vi "Helium Test - Step 5.vi"(7 "Step":i32, 8 "error in":errorcluster, 9 "Test Results In":T9, 10 "Gas":T8, 11 "Test Configuration":T1) -> (0 "error out":errorcluster, 1 "Test Results Out":T9, 2 "Gas Out":T8 caption="Gas", 3 "Test Configuration Out":T1)   [LabVIEW 2015]
uses:
  CAN Communication/PAS/Typedefs/Session Handle.ctl
  CAN Communication/PAS/PAS.lvclass
  Controls/Test Results.ctl
  Controls/Step Result.ctl
  Controls/Test Configuration.ctl
  Controls/Vacuum Test.ctl
  Controls/Test Timing.ctl
  Controls/Vaccum Thresholds.ctl
  Controls/Helium Test.ctl
  Controls/Helium Thresholds.ctl
  Controls/Functional Test.ctl
  CAN Communication/PAS/Typedefs/Valves.ctl
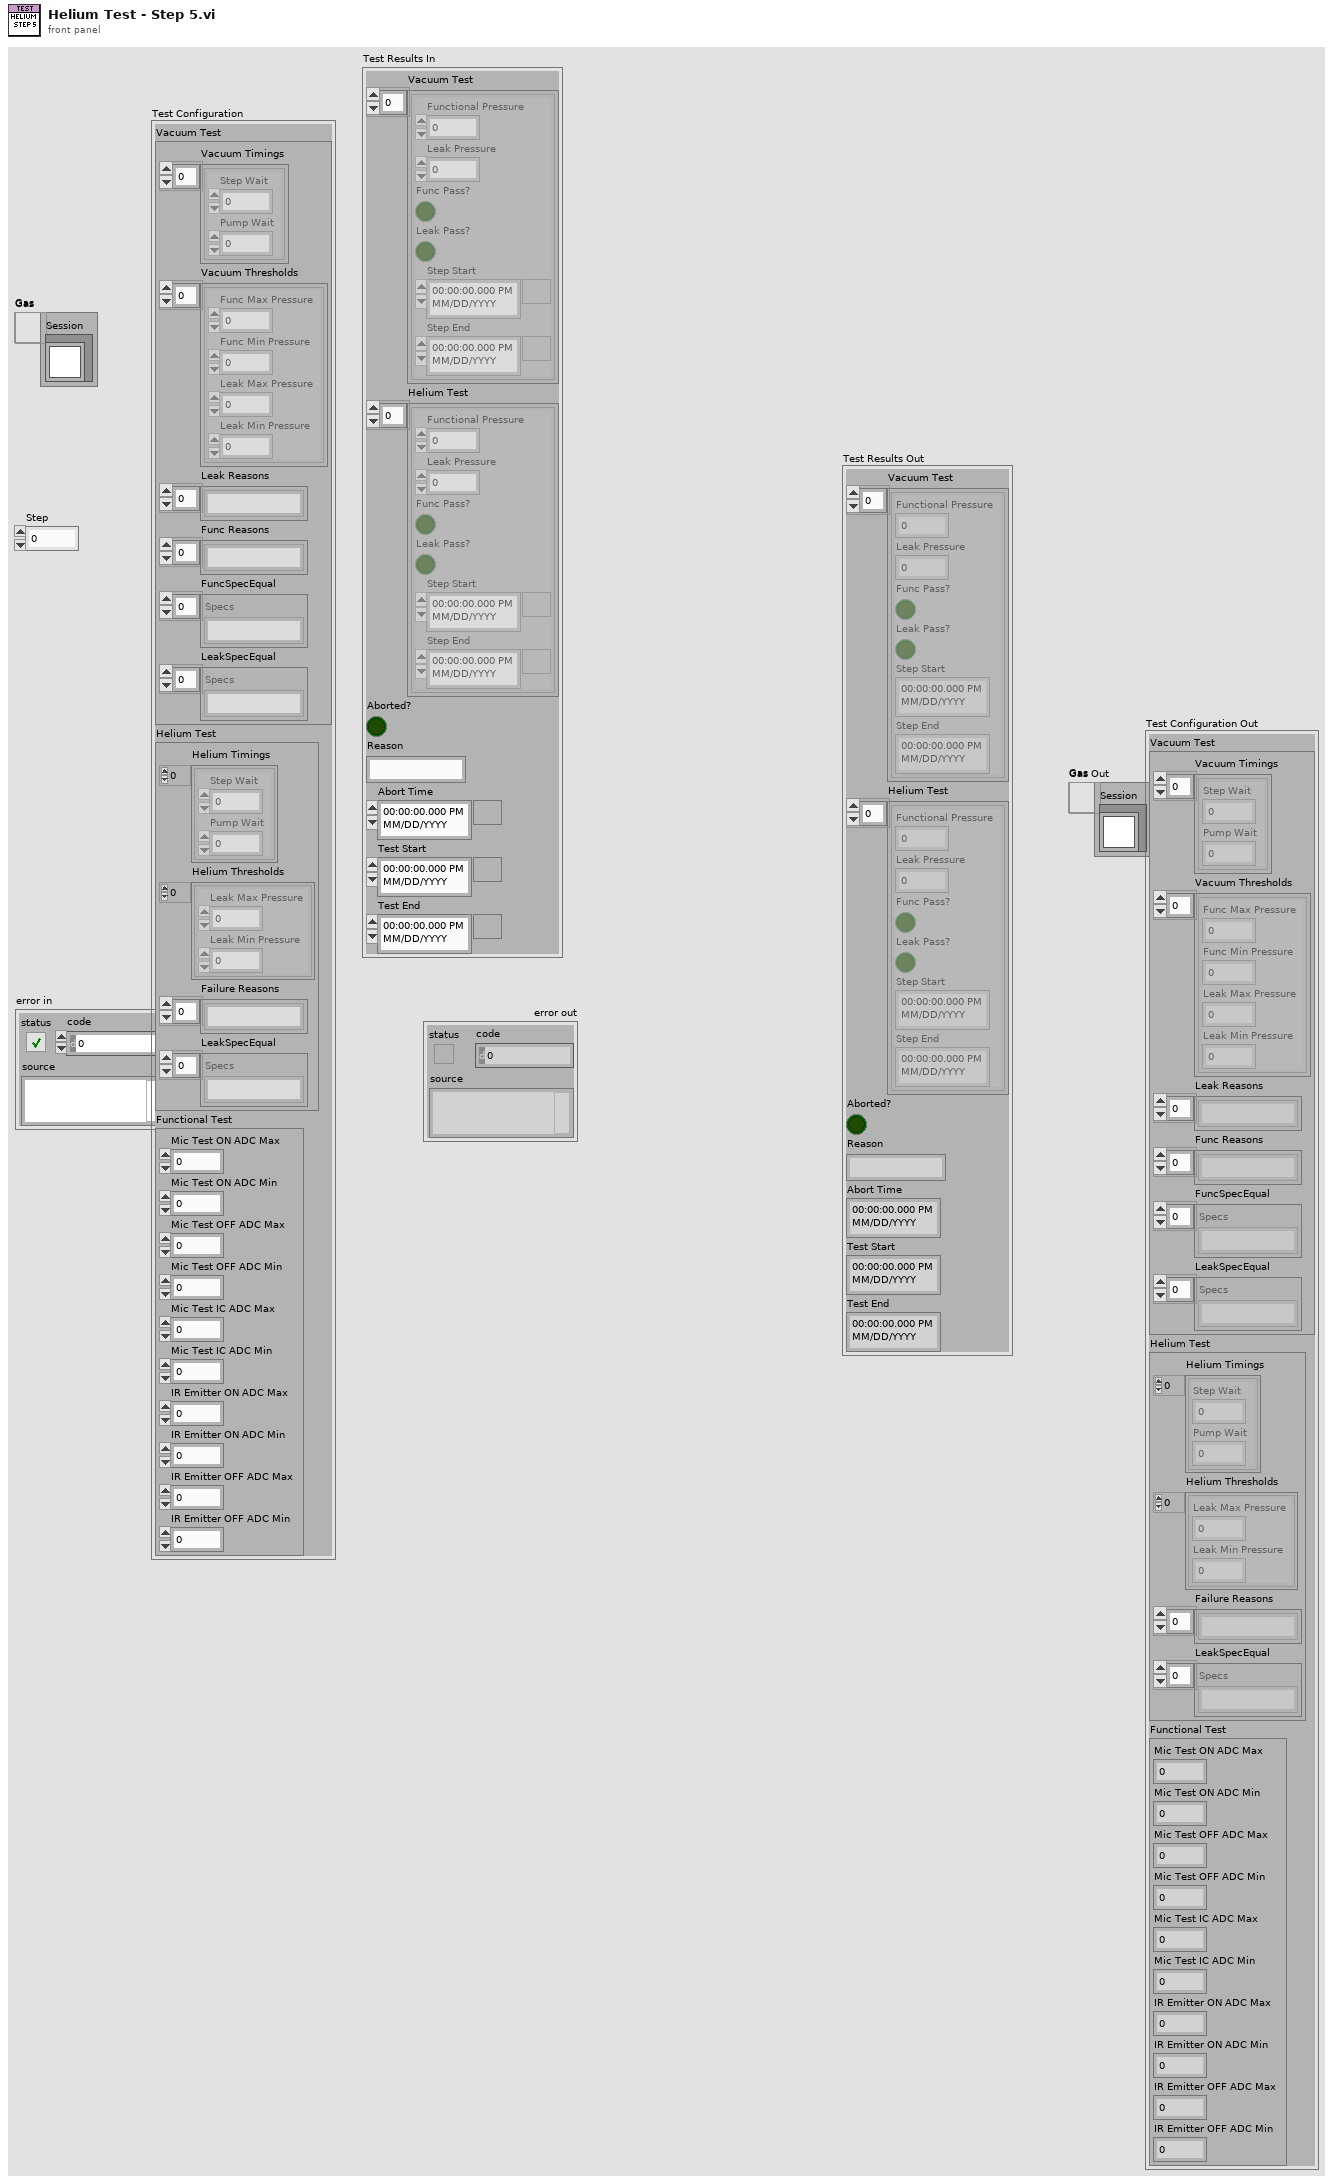
[diagram p1: front panel]
types:
  T1 = typedef "Test Configuration.ctl" = cluster{"Vacuum Test":T2, "Helium Test":T5, "Functional Test":T7}
  T2 = typedef "Vacuum Test.ctl" = cluster{"Vacuum Timings":T3[], "Vacuum Thresholds":T4[], "Leak Reasons":string[], "Func Reasons":string[], "FuncSpecEqual":string[], "LeakSpecEqual":string[]}
  T3 = typedef "Test Timing.ctl" = cluster{"Step Wait":dbl, "Pump Wait":dbl}
  T4 = typedef "Vaccum Thresholds.ctl" = cluster{"Func Max Pressure":dbl, "Func Min Pressure":dbl, "Leak Max Pressure":dbl, "Leak Min Pressure":dbl}
  T5 = typedef "Helium Test.ctl" = cluster{"Helium Timings":T3[], "Helium Thresholds":T6[], "Failure Reasons":string[], "LeakSpecEqual":string[]}
  T6 = typedef "Helium Thresholds.ctl" = cluster{"Leak Max Pressure":dbl, "Leak Min Pressure":dbl}
  T7 = typedef "Functional Test.ctl" = cluster{"Mic Test ON ADC Max":dbl, "Mic Test ON ADC Min":dbl, "Mic Test OFF ADC Max":dbl, "Mic Test OFF ADC Min":dbl, "Mic Test IC ADC Max":dbl, "Mic Test IC ADC Min":dbl, "IR Emitter ON ADC Max":dbl, "IR Emitter ON ADC Min":dbl, "IR Emitter OFF ADC Max":dbl, "IR Emitter OFF ADC Min":dbl}
  T8 = typedef "PAS.lvclass/Session Handle.ctl" = refnum<data-value>
  T9 = typedef "Test Results.ctl" = cluster{"Vacuum Test":T10[], "Helium Test":T10[], "Aborted?":bool, "Reason":string, "Abort Time":timestamp, "Test Start":timestamp, "Test End":timestamp}
  T10 = typedef "Step Result.ctl" = cluster{"Functional Pressure":dbl, "Leak Pressure":dbl, "Func Pass?":bool, "Leak Pass?":bool, "Step Start":timestamp, "Step End":timestamp}
  T11 = typedef "PAS.lvclass/Valves.ctl" = u16
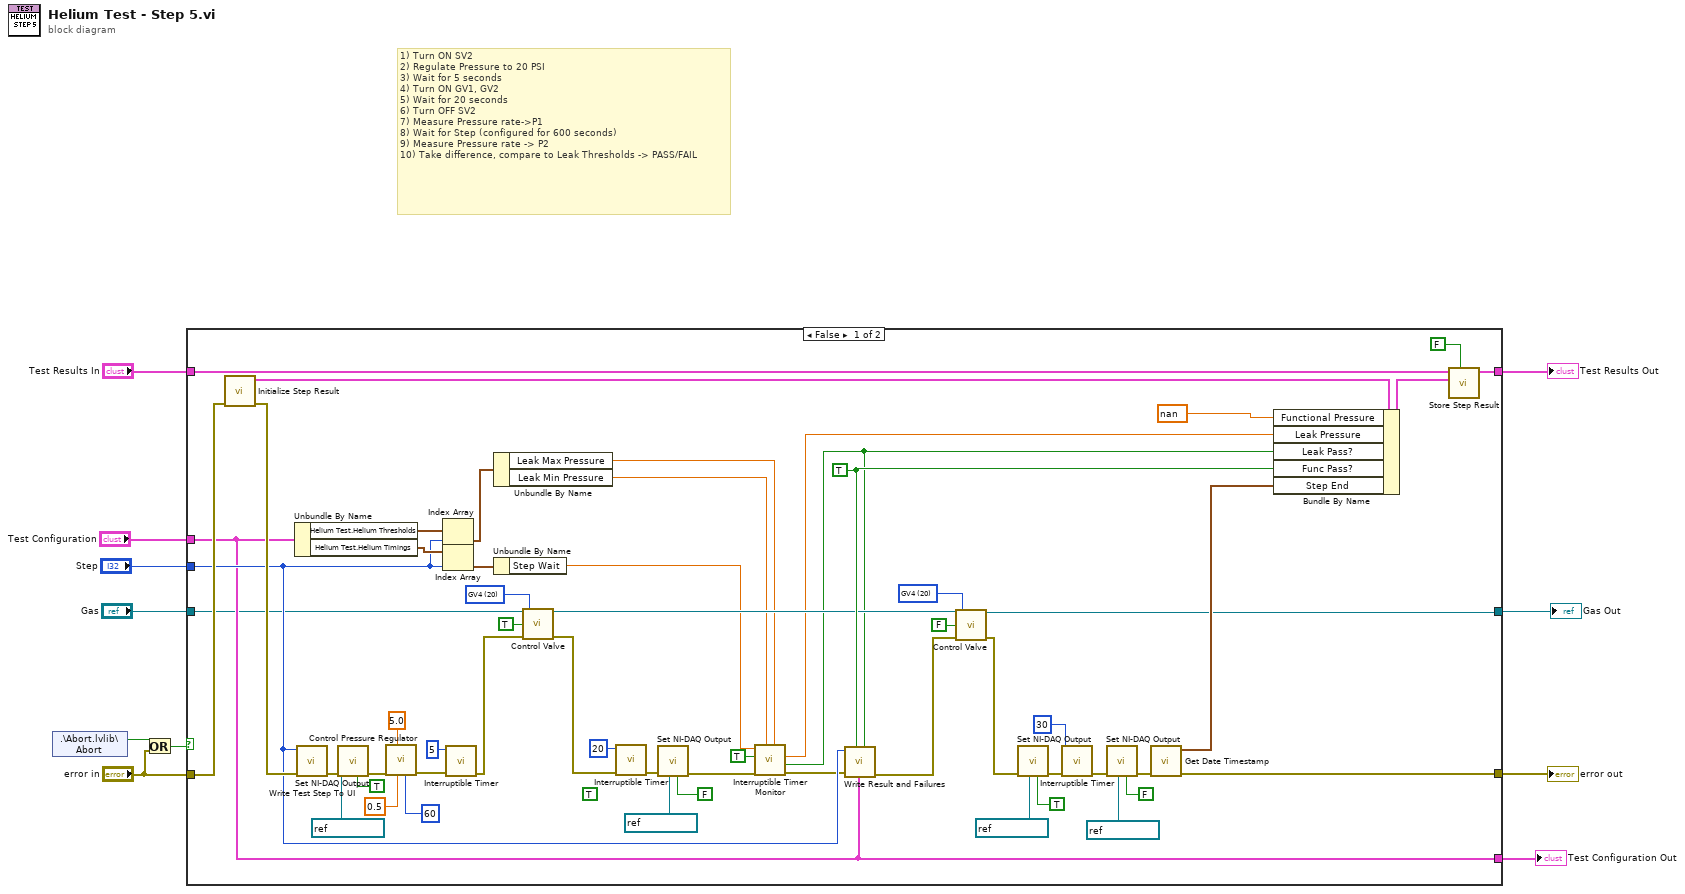
[diagram p0: block diagram]
diagram:
  # "1) Turn ON SV2\n2) Regulate Pressure to 20 PSI\n3) Wait for 5 seconds\n4) Turn ON GV1, GV2\n5) Wait for 20 seconds\n6) Turn OFF SV2\n7) Measure Pressure rate->P1\n8) Wait for Step (configured for 600 seconds)\n9) Measure Pressure rate -> P2\n10) Take difference, compare to Leak Thresholds -> PASS/FAIL"
  n1 = shared-variable ".\\Abort.lvlib\\Abort"() -> (w10:bool)  [unwired: 1 in, 1 out]
  n2 = Or(x=w10, y="error in") -> (x .or. y?=w9:bool)
  n3 = case shown="False" w9 {
    tunnel: "error in" -> [w68 w71]
    tunnel: "Test Results In" -> [w65 w72]
    tunnel: [w66 w72] -> w7
    tunnel: [w12 w71] -> w6
    tunnel: "Test Configuration" -> [w56 w70]
    tunnel: "Step" -> [w57 _]
    tunnel: [w56 w70] -> w1
    tunnel: [w34 w69] -> w3
    tunnel: "Gas" -> [w42 w69]
    frame False {
      w36 = T11 20 items=["GV1"=17, "GV2"=18, "GV3"=19, "GV4"=20] ("Valves")
      w41 = T11 20 items=["GV1"=17, "GV2"=18, "GV3"=19, "GV4"=20] ("Valves")
      (unwired) TRUE ("State")
      w54 = TRUE ("Func Pass?")
      n4 = call "Initialize Step Result.vi"("error in (no error)"=w68) -> ("error out"=w67:errorcluster, "New Step Result"=w64:T10)  [unwired: 8 in, 1 out]
      n5 = Unbundle By Name(w56) -> ("Helium Test.Helium Thresholds"=w61:T6[], "Helium Test.Helium Timings"=w60:T3[])
      n6 = call "Write Test Step To UI.vi"("error in (no error)"=w67, "Step"=w57) -> ("error out"=w48:errorcluster)  [unwired: 9 in]
      n7 = call "Set NI-DAQ Output.vi"("State"=TRUE, "Channel"=refnum<k21> "SV2_PAS", "error in (no error)"=w48) -> ("error out"=w51:errorcluster)  [unwired: 8 in]
      n8 = call "Control Pressure Regulator.vi"("Timeout"=60, "y"=0.5, "error in"=w51, "Desired PSI"=5.0) -> ("error out"=w49:errorcluster)  [unwired: 6 in, 1 out]
      n9 = Index Array(array=w61, index=w57) -> (element=w58:T6)
      n10 = Index Array(array=w60, index=w57) -> (element=w59:T3)
      n11 = call "Interruptible Timer.vi"("error in (no error)"=w49, "Wait (s)"=5) -> ("error out"=w39:errorcluster)  [unwired: 7 in, 2 out]
      n12 = Unbundle By Name(w58) -> ("Leak Max Pressure"=w19:dbl, "Leak Min Pressure"=w20:dbl)
      n13 = Unbundle By Name(w59) -> ("Step Wait"=w22:dbl)
      n14 = call "Control Valve.vi"("Session Handle in"=w42, "Valves"=w41, "Energize?"=TRUE, "error in (no error)"=w39) -> ("Session Handle out"=w35:T8, "error out"=w38:errorcluster)  [unwired: 8 in, 2 out]
      n15 = call "Interruptible Timer.vi"("error in (no error)"=w38, "Wait (s)"=20) -> ("error out"=w45:errorcluster)  [unwired: 7 in, 2 out]
      n16 = call "Set NI-DAQ Output.vi"("State"=FALSE, "Channel"=refnum<k21> "SV2_PAS", "error in (no error)"=w45) -> ("error out"=w23:errorcluster)  [unwired: 8 in]
      n17 = call "Interruptible Timer Monitor.vi"("Max"=w19, "Min"=w20, "error in (no error)"=w23, "Update UI?"=TRUE, "Wait (s)"=w22) -> ("error out"=w14:errorcluster, "In Range?"=w16:bool, "Leak Rate"=w18:dbl)  [unwired: 3 in, 1 out]
      n18 = call "Write Result and Failures.vi"("Leak"=w16, "Test Configuration"=w56, "Func"=w54, "error in (no error)"=w14, "Step"=w57) -> ("error out"=w13:errorcluster)  [unwired: 6 in]
      n19 = call "Control Valve.vi"("Session Handle in"=w35, "Valves"=w36, "Energize?"=FALSE, "error in (no error)"=w13) -> ("Session Handle out"=w34:T8, "error out"=w26:errorcluster)  [unwired: 8 in, 2 out]
      n20 = call "Set NI-DAQ Output.vi"("State"=TRUE, "Channel"=refnum<k21> "SV1_PAS", "error in (no error)"=w26) -> ("error out"=w33:errorcluster)  [unwired: 8 in]
      n21 = call "Interruptible Timer.vi"("error in (no error)"=w33, "Wait (s)"=30) -> ("error out"=w30:errorcluster)  [unwired: 7 in, 2 out]
      n22 = call "Set NI-DAQ Output.vi"("State"=FALSE, "Channel"=refnum<k21> "SV1_PAS", "error in (no error)"=w30) -> ("error out"=w25:errorcluster)  [unwired: 8 in]
      n23 = call "Get Date Timestamp.vi"("error in (no error)"=w25) -> ("error out"=w12:errorcluster, "current time"=w62:timestamp)  [unwired: 9 in]
      n24 = Bundle By Name(cluster=w64, "Functional Pressure"=nan, "Leak Pressure"=w18, "Leak Pass?"=w16, "Func Pass?"=w54, "Step End"=w62) -> (w63:T10)
      n25 = call "Store Step Result.vi"("Vacuum?"=FALSE, "Step Result"=w63, "Test Results In"=w65) -> ("Test Results Out"=w66:T9)  [unwired: 8 in]
    }
    frame True {
    }
  }
  "error out" <- w6
  "Test Results Out" <- w7
  "Gas Out" <- w3
  "Test Configuration Out" <- w1
